vi "Intan_mainControlPanel_64chan_ambulatory.vi"() -> ()   [LabVIEW 2017]
panel:
  out "ADC calib":bool
  in  "Config Hardware Filter":bool=TRUE
  in  "ConfigReg [0:7, aPwr]":bool=TRUE
  in  "R_L source":u8(ring)=1 items=["ON-chip", "OFF-chip"]
  in  "Lower cutoff":u8(ring)=12 items=["10 Hz", "7.5 Hz", "5.0 Hz", "3.0 Hz", "2.5 Hz", "2.0 Hz", "1.5 Hz", "1.0 Hz", "0.75 Hz", "0.5 Hz", "0.3 Hz", "0.25 Hz", "0.10 Hz"]
  in  "Upper cutoff":u8(ring)=12 items=["5.0 kHz", "3.0 kHz", "2.5 kHz", "2.0 kHz", "1.5 kHz", "1.0 kHz", "750 Hz", "500 Hz", "300 Hz", "250 Hz", "200 Hz", "150 Hz", "100 Hz"]
  out "DT strea, (us)":dbl
  out "actual rate  (Hz)":dbl
  in  "UART Stream  Rate (Hz)":u16=200
  out "DT samp (us)":dbl
  out "actual fs (Hz)":dbl
  in  "Desired Fs (Hz)":u16=200
  in  "Save to SD card":bool=TRUE
  in  "SD card File Name":string
  out "Serial Port Type":string
  in  "VISA resource name":refnum<visa-resource-name>="COM33"
  in  "Start Data Stream":bool
  out "HeaderFilePath":path
  in  "Save Display Data":bool
  out "Config Result":string
  out "Teensy response":string
  out "Raw data file path":path
  in  "Save Raw Data":bool=TRUE
  # "Intan-Teensy Bioelectric Module: \nconfigure hardware and serial port \nAmbulatory 64 chan"
  # "Configure all settings, then click run arrow.\n\nWhen config is complete, click the purple\nbutton to start data stream.\n\nSeparate VI will pop open to display signals"
  # "TODO 01 May 2017 JE\n\nSTATUS: Operational, beta.\n\nSOFTWARE issues:\n\n - Set decimation ratio to ensure Nsamps in display never exceeds chart limit\nor sensible human visibility bound (for now set chart history length = 50000.\nFor typical max sampling rates of 500 Hz in our applications, this still allows up to 100 s\nof data display (ridiculously long).  In practice, could probably increase performance\nby decreasing chart history to something smaller like 20000.\n\n\n- Make bdf style header and write to file (low priority)\n\n -  Stream to main fig window, Present only does this in subVI (IntanStream_Parallel Loops.vi)\n  SOLN: just pop open subVI automatically when called, but pre-set filters (?)\n\nHARDWARE issues: \n\n\nNeed to gracefully recover when data sync is lost. Option to reboot Teensy and recover connection? \nCurrent error checking not working, don' know why.  Software reset tricky to implement:\nhttps://forum.pjrc.com/archive/index.php/t-24304.html\nBest solution for now, unplug then replug power.  This puts Teensy back into initial state.\n\n-Option to stream subset of channels.  This will allow higher data rate for wireless streaming, if desired."
  # "Intan Amp Config"
  # "Hardware Filter Settings"
  # "UART streaming"
  # "ADC Sampling"
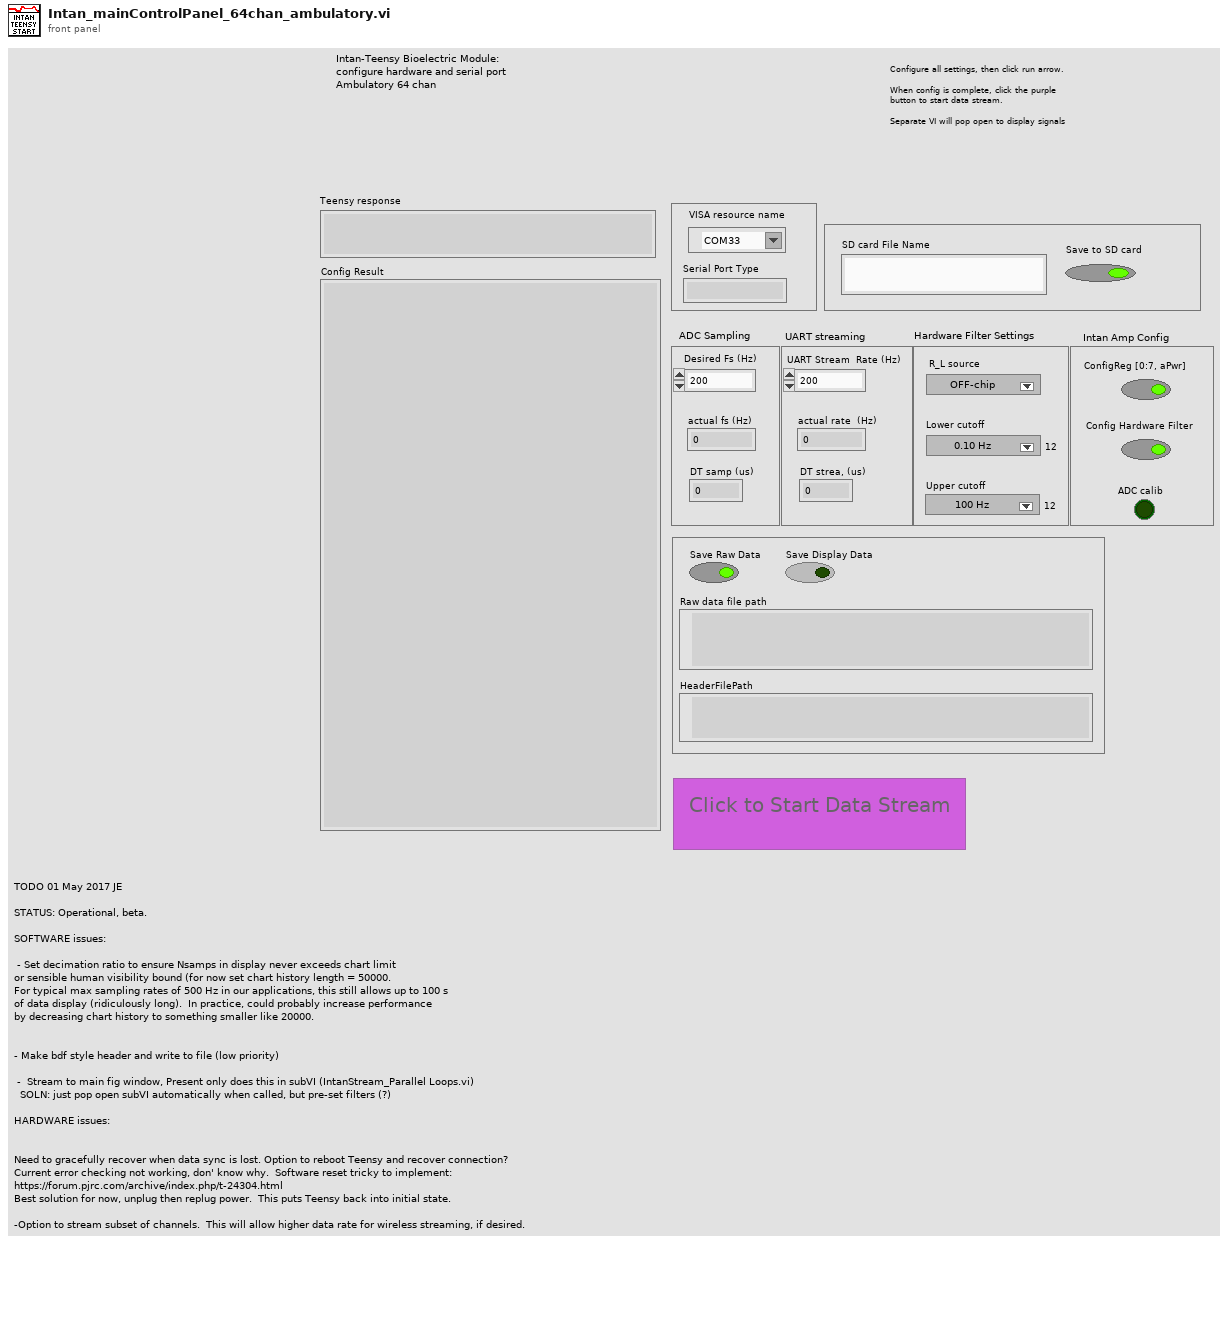
[diagram p1: front panel]
types:
  T1 = enum8{"Enabled", "Disabled", "Disabled and Grayed Out"}
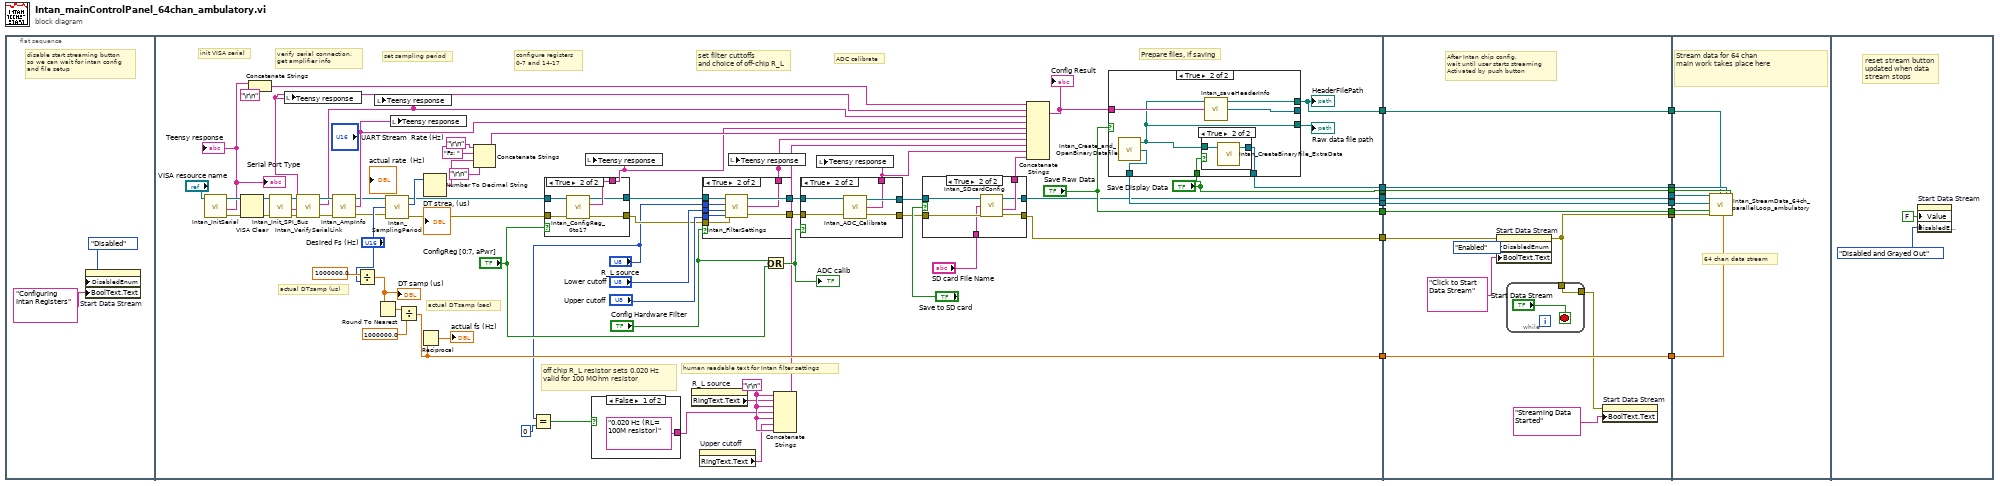
[diagram p0: block diagram]
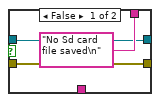
[diagram p2: hidden frame]
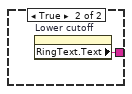
[diagram p3: hidden frame]
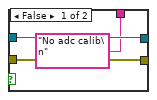
[diagram p4: hidden frame]
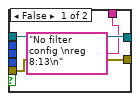
[diagram p5: hidden frame]
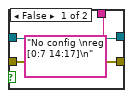
[diagram p6: hidden frame]
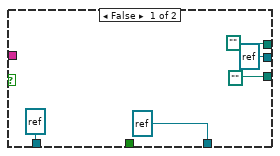
[diagram p7: hidden frame]
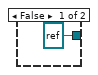
[diagram p8: hidden frame]
diagram:
  n1 = flat-sequence {
    tunnel: [w79] -> w10
    tunnel: [w67] -> w9
    tunnel: [w64] -> w8
    tunnel: ["Save Raw Data"] -> w7
    tunnel: ["Save Display Data"] -> w6
    tunnel: [w23] -> w5
    tunnel: [w45] -> w2
    tunnel: [w21] -> w1
    tunnel: [w144] -> w16
    tunnel: [w150] -> w15
    tunnel: [w149] -> w14
    tunnel: [w148] -> w13
    tunnel: [w147] -> w12
    tunnel: [w146] -> w11
    tunnel: w6 -> [w146]
    tunnel: w7 -> [w147]
    tunnel: w8 -> [w148]
    tunnel: w9 -> [w149]
    tunnel: w10 -> [w150]
    tunnel: w5 -> [w143]
    tunnel: [w142] -> w4
    tunnel: [w141] -> w3
    tunnel: w2 -> [w141]
    tunnel: w1 -> [w142]
    tunnel: w16 -> [w157]
    tunnel: w15 -> [w155]
    tunnel: w14 -> [w160]
    tunnel: w13 -> [w158]
    tunnel: w12 -> [w156]
    tunnel: w11 -> [w159]
    tunnel: w4 -> [w154]
    tunnel: w3 -> [w153]
    frame #0 {
      # "disable start streaming button\nso we can wait for intan config\nand file setup"
      n2 = property on="Start Data Stream" class="Bool (strict)"("DisabledEnum"=T1."Disabled" ("Disabled"), "BoolText.Text"="Configuring Intan Registers" ("Boolean Text.Text")) -> ()  [unwired: 2 in, 2 out]
    }
    frame #1 {
      w40 = "\r\n"
      # "off chip R_L resistor sets 0.020 Hz \nvalid for 100 MOhm resistor"
      # "human readable text for Intan filter settings"
      # "Prepare files, if saving"
      # "ADC calibrate"
      # "set filter cuttoffs \nand choice of off-chip R_L"
      # "configure registers\n0-7 and 14-17"
      # "set sampling period"
      # "verify serial connection,\nget amplifier info"
      # "init VISA serial"
      # "actual DTsamp (sec)"
      # "actual DTsamp (us)"
      n3 = call "Intan_InitSerial.vi"("VISA resource name"="VISA resource name") -> ("VISA resource name out"=w44:refnum<visa-resource-name>, "Text response"=w42:string, "error out"=w78:errorcluster)  [unwired: 3 in]
      "Teensy response" <- w42
      "Serial Port Type" <- w42
      n4 = VISA Clear(VISA resource name=w44, error in (no error)=w78) -> (VISA resource name out=w31:refnum<visa-resource-name>, error out=w30:errorcluster)
      n5 = Concatenate Strings(w42, "\r\n") -> (w27:string)
      n6 = call "Intan_Init_SPI_Bus.vi"("error in"=w30, "VISA resource name"=w31) -> ("error out"=w29:errorcluster, "Text response"=w26:string, "VISA resource name out"=w28:refnum<visa-resource-name>)  [unwired: 3 in]
      n7 = local write "Teensy response"(w26) -> ()
      n8 = call "Intan_VerifySerialLink.vi"("error in"=w29, "VISA resource name"=w28) -> ("error out"=w80:errorcluster, "Text response"=w76:string, "VISA resource name out"=w81:refnum<visa-resource-name>)  [unwired: 7 in]
      n9 = call "Intan_AmpInfo.vi"("error in"=w80, "VISA resource name"=w81) -> ("error out"=w60:errorcluster, "Text response"=w77:string, "VISA resource name out"=w61:refnum<visa-resource-name>)  [unwired: 1 in]
      n10 = Divide(x=1000000.0, y="Desired Fs (Hz)") -> (x/y=w46:dbl)
      "DT samp (us)" <- w46
      n11 = local write "Teensy response"(w76) -> ()
      n12 = Round To Nearest(number=w46) -> (nearest integer value=w69:dbl)
      n13 = call "Intan_SamplingPeriod.vi"("VISA resource name"=w61, "Desired Fs (Hz)"="Desired Fs (Hz)", "error in"=w60) -> ("VISA resource name out"=w59:refnum<visa-resource-name>, "FS actual (Hz)"=w75:i32, "error out"=w58:errorcluster)  [unwired: 1 out]
      n14 = local write "Teensy response"(w77) -> ()
      n15 = Divide(x=w69, y=1000000.0 ("x")) -> (x/y=w67:dbl)
      n16 = Reciprocal(x=w67) -> (1/x=→"actual fs (Hz)":dbl)
      n17 = Number To Decimal String(number=w75) -> (decimal integer string=w74:string)  [unwired: 1 in]
      n18 = Concatenate Strings("\r\n", "Fs: " ("string"), w74, "\r\n") -> (w72:string)
      n19 = Equal?(x="R_L source", y=u8 0) -> (x = y?=w35:bool)
      n20 = case shown="True" "ConfigReg [0:7, aPwr]" {
        tunnel: w59 -> [w116 w122]
        tunnel: w58 -> [w115 w121]
        tunnel: ["No config \nreg [0:7 14:17]\n" ("Text response") w120] -> w57
        tunnel: [w116 w119] -> w54
        tunnel: [w115 w118] -> w53
        frame False {
        }
        frame True {
          n21 = call "Intan_ConfigReg_0to17.vi"("error in"=w121, "VISA resource name"=w122) -> ("error out"=w118:errorcluster, "Text response"=w120:string, "VISA resource name out"=w119:refnum<visa-resource-name>)  [unwired: 7 in]
        }
      }
      n22 = local write "Teensy response"(w57) -> ()
      n23 = case shown="False" w35 {
        tunnel: ["0.020 Hz (RL= 100M resistor)" ("string") w95] -> w33
        frame False {
        }
        frame True {
          n24 = property on="Lower cutoff" class="Ring (strict)"() -> ("RingText.Text"=w95:string)  [unwired: 2 in, 2 out]
        }
      }
      n25 = property on="R_L source" class="Ring (strict)"() -> ("RingText.Text"=w38:string)  [unwired: 2 in, 2 out]
      n26 = property on="Upper cutoff" class="Ring (strict)"() -> ("RingText.Text"=w39:string)  [unwired: 2 in, 2 out]
      n27 = case shown="True" "Config Hardware Filter" {
        tunnel: "R_L source" -> [_ w114]
        tunnel: "Lower cutoff" -> [_ w113]
        tunnel: "Upper cutoff" -> [_ w112]
        tunnel: w54 -> [w106 w111]
        tunnel: w53 -> [w105 w110]
        tunnel: [w106 w109] -> w52
        tunnel: [w105 w108] -> w51
        tunnel: ["No filter config \nreg 8:13\n" ("Text response") w107] -> w50
        frame False {
        }
        frame True {
          n28 = call "Intan_FilterSettings.vi"("VISA resource name"=w111, "R_L source"=w114, "Lower cutoff"=w113, "Upper cutoff"=w112, "error in"=w110) -> ("VISA resource name out"=w109:refnum<visa-resource-name>, "Text response"=w107:string, "error out"=w108:errorcluster)
        }
      }
      n29 = local write "Teensy response"(w50) -> ()
      n30 = Or(x="Config Hardware Filter", y="ConfigReg [0:7, aPwr]") -> (x .or. y?=w49:bool)
      "ADC calib" <- w49
      n31 = Concatenate Strings(w40, w38, w40, w33, w40, w39, w40) -> (w36:string)
      n32 = case shown="True" w49 {
        tunnel: w52 -> [w98 w103]
        tunnel: w51 -> [w97 w102]
        tunnel: [w97 w101] -> w22
        tunnel: [w98 w100] -> w20
        tunnel: ["No adc calib\n" ("Text response") w99] -> w37
        frame False {
        }
        frame True {
          n33 = call "Intan_ADC_Calibrate.vi"("error in"=w102, "VISA resource name"=w103) -> ("error out"=w101:errorcluster, "Text response"=w99:string, "VISA resource name out"=w100:refnum<visa-resource-name>)  [unwired: 1 in]
        }
      }
      n34 = local write "Teensy response"(w37) -> ()
      n35 = case shown="True" "Save to SD card" {
        tunnel: ["No Sd card file saved\n" ("Text response") w93] -> w24
        tunnel: [w85 w92] -> w23
        tunnel: w22 -> [w85 w91]
        tunnel: w20 -> [w86 w90]
        tunnel: [w86 w89] -> w21
        tunnel: "SD card File Name" -> [_ w88]
        frame False {
        }
        frame True {
          n36 = call "Intan_SDcardConfig.vi"("VISA resource name"=w90, "SdFilename"=w88, "error in"=w91) -> ("VISA resource name out"=w89:refnum<visa-resource-name>, "Return File Name"=w93:string, "error out"=w92:errorcluster)  [unwired: 1 out]
        }
      }
      n37 = Concatenate Strings(w27, w26, w76, w77, w57, w72, w50, w36, w37, w24) -> (w65:string)
      "Config Result" <- w65
      n38 = case shown="True" "Save Raw Data" {
        tunnel: [refnum<file> refnum ("refnum out") w134] -> w79
        tunnel: w65 -> [_ w133]
        tunnel: [refnum<file> refnum ("refnum out") w132] -> w64
        tunnel: "Save Display Data" -> [_ w131]
        tunnel: [path "" w130] -> w45
        tunnel: [path "" w129] -> w55
        tunnel: [refnum<file> refnum ("hdr_file_ref_num_out") w128] -> _
        frame False {
        }
        frame True {
          n39 = call "Intan_Create_and_OpenBinaryDatafile.vi"() -> ("file path"=w129:path, "refnum out"=w134:refnum<file>)  [unwired: 2 in, 1 out]
          n40 = case shown="True" w131 {
            tunnel: w129 -> [_ w137]
            tunnel: [refnum<file> refnum ("refnum out") w136] -> w132
            frame False {
            }
            frame True {
              n41 = call "Intan_CreateBinaryFile_ExtraData.vi"("DataFilePath"=w137) -> ("refnum out"=w136:refnum<file>)  [unwired: 3 in, 1 out]
            }
          }
          n42 = call "Intan_saveHeaderInfo.vi"("header text"=w133, "DataFilePath"=w129) -> ("hdr_file_ref_num_out"=w128:refnum<file>, "HeaderFilePath"=w130:path)  [unwired: 1 in, 1 out]
        }
      }
      "HeaderFilePath" <- w45
      "Raw data file path" <- w55
    }
    frame #2 {
      # "After Intan chip config,\nwait until user starts streaming\nActivated by push button"
      n43 = property on="Start Data Stream" class="Bool (strict)"(error in=w143, "DisabledEnum"=T1."Enabled" ("Disabled"), "BoolText.Text"="Click to Start Data Stream" ("Boolean Text.Text")) -> (error out=w144:errorcluster)  [unwired: 1 in, 1 out]
      n44 = while {
        tunnel: w144 -> [w151]
        tunnel: [w151] -> w139
        stop <- "Start Data Stream" stop-if-true
      }
      n45 = property on="Start Data Stream" class="Bool (strict)"(error in=w139, "BoolText.Text"="Streaming Data Started" ("Boolean Text.Text")) -> ()  [unwired: 1 in, 2 out]
    }
    frame #3 {
      # "64 chan data stream"
      # "Stream data for 64 chan\nmain work takes place here"
      n46 = call "Intan_StreamData_64ch_parallelLoop_ambulatory.vi"("VISA resource name"=w154, "refnum in"=w155, "Save Binary Data"=w156, "error in"=w157, "hdr fpath"=w153, "DT_scale (sec)"=w160, "aux file ref num"=w158, "save aux file"=w159) -> ()  [unwired: 8 in, 4 out]
    }
    frame #4 {
      # "reset stream button \nupdated when data\nstream stops"
      n47 = property on="Start Data Stream" class="Bool (strict)"("Value"=FALSE ("Start Data Stream"), "DisabledEnum"=T1."Disabled and Grayed Out" ("Disabled")) -> ()  [unwired: 2 in, 2 out]
    }
  }
